vi "Coordinate_Trans_.vi"(0 "Input Position":dbl[](array[numeric])=[0.0, 0.0, 0.0] format="%.2f") -> (1 "X":dbl, 2 "Y":dbl, 3 "Z":dbl)   [LabVIEW 2010]
uses:
  Globals/Trav_pos_global.vi
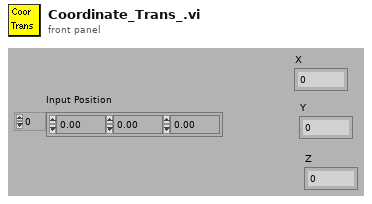
[diagram p1: front panel]
types:
  T1 = typedef "Tunnel_Coordinates.ctl" = enum16{"Work in Tunnel Coordinates", "Work in Model Coordinates"}
  T2 = enum16{"To Traverse Coordinates", "To User Coordinates"}
  T3 = cluster{"Output Position[0]":dbl, "Output Position[1]":dbl, "Output Position[2]":dbl}
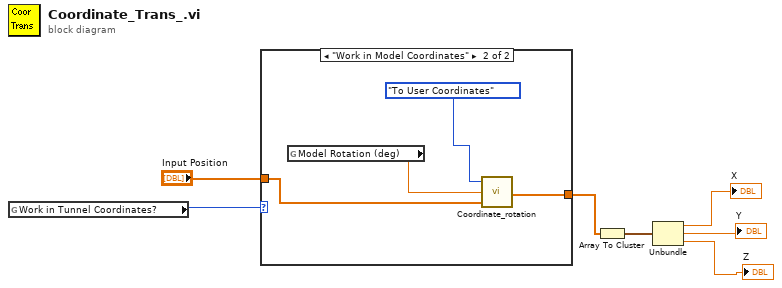
[diagram p0: block diagram]
diagram:
  n1 = global read "Trav_pos_global.vi" "Work in Tunnel Coordinates?"() -> (w6:T1)
  n2 = case shown="\"Work in Model Coordinates\"" w6 {
    tunnel: [w8 w10] -> w4
    tunnel: "Input Position" -> [w8 w11]
    frame "Work in Tunnel Coordinates" {
    }
    frame "Work in Model Coordinates" {
      n3 = global read "Trav_pos_global.vi" "Model Rotation (deg)"() -> (w9:dbl)
      n4 = call "Coordinate_rotation.vi"("Input Position"=w11, "Coordinate rotation (deg)"=w9, "Mode"=T2."To User Coordinates") -> ("Output Position"=w10:dbl[])
    }
  }
  n5 = Array To Cluster(array=w4) -> (cluster=w5:T3)
  n6 = Unbundle(w5) -> ("Output Position[0]"=→"X":dbl, "Output Position[1]"=→"Y":dbl, "Output Position[2]"=→"Z":dbl)
